vi "AB_820_850_Project_Source_VI.vi"(6 "dataForPrevious":T1, 7 "action":T6, 8 "error in (no error)":errorcluster, 9 "index in":i32, 10 "dataSource in":T5, 11 "buildObject":T4) -> (0 "error out":errorcluster, 1 "index out":i32, 2 "dataSource out":T5, 3 "buildObject out":T4)   [LabVIEW 2020]
doc: "Reads and writes the data to the object property bag."
uses:
  <resource>/Framework/Providers/API/ItemRef.ctl
  <vilib>/AppBuilder/RW_Project/AB_RW_Project_PropBag_Action.ctl
  <vilib>/AppBuilder/RW_Project/AB_RW_Project_Source_Data_for_Previous.ctl
  <vilib>/AppBuilder/AB_BuildType.ctl
  <vilib>/Utility/lvfile.llb/LVFileType.ctl
  <vilib>/Utility/lvfile.llb/NI_FileType.lvlib
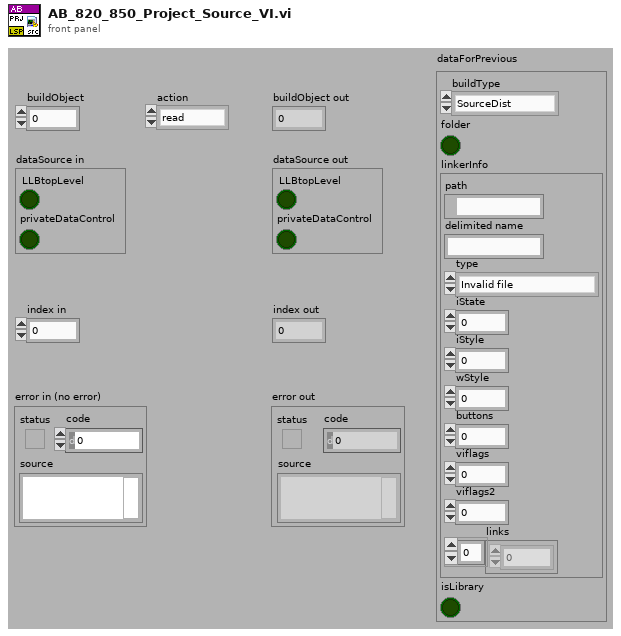
[diagram p1: front panel]
types:
  T1 = typedef "AB_RW_Project_Source_Data_for_Previous.ctl" = cluster{"buildType":T2, "folder":bool, "linkerInfo":cluster{"path":path, "delimited name":string, "type":T3, "iState":u32, "iStyle":u16, "wStyle":u16, "buttons":u16, "viflags":u32, "viflags2":u32, "links":u32[]}, "isLibrary":bool}
  T2 = typedef "AB_BuildType.ctl" = enum16{"SourceDist", "EXE", "DLL", "RTExe"}
  T3 = typedef "NI_FileType.lvlib/LVFileType.ctl" = enum32{"Invalid file", "Unknown type", "Instrument", "Control", "Polymorphic VI", "Project", "Library", "LVClass", "XControl", "XNode", "Shared library", ".NET assembly", "ActiveX interface", "CIN", "Run-time menu", "Palette menu", "Help file", "LLB", "XNode Edit Dependency", "Class Private Data Control", "Statechart", "MathScript .m file", "Ladder Diagram", "LVLibp", "XNode Build Dependency"}
  T4 = typedef "ItemRef.ctl" = u64
  T5 = cluster{"LLBtopLevel":bool, "privateDataControl":bool}
  T6 = typedef "AB_RW_Project_PropBag_Action.ctl" = enum16{"read", "write", "clear", "readPrevious", "writePrevious", "clearPrevious"}
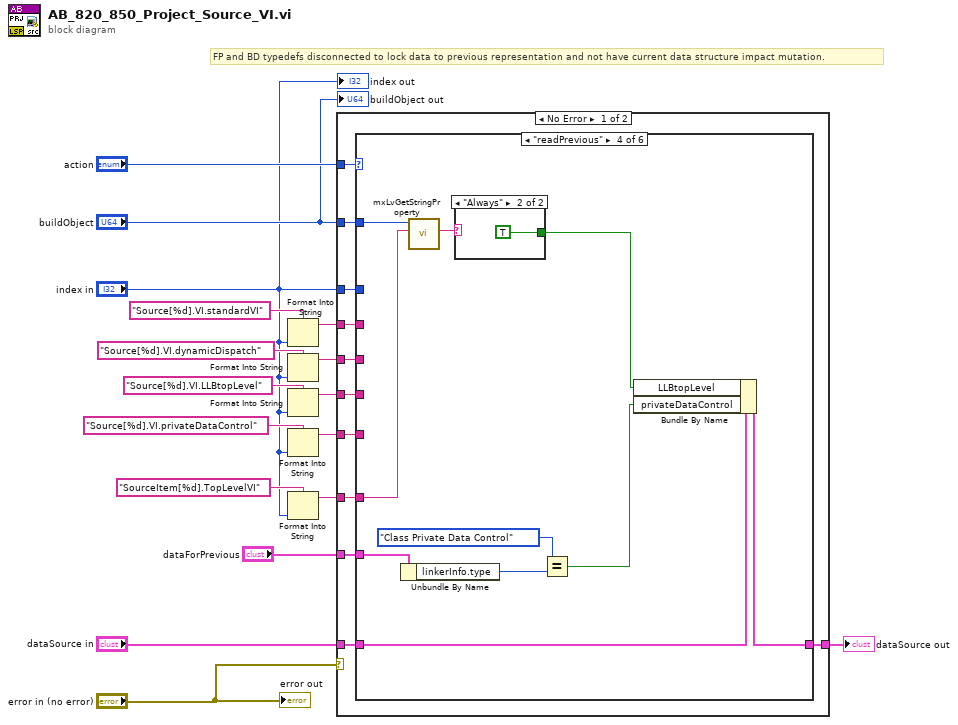
[diagram p0: block diagram]
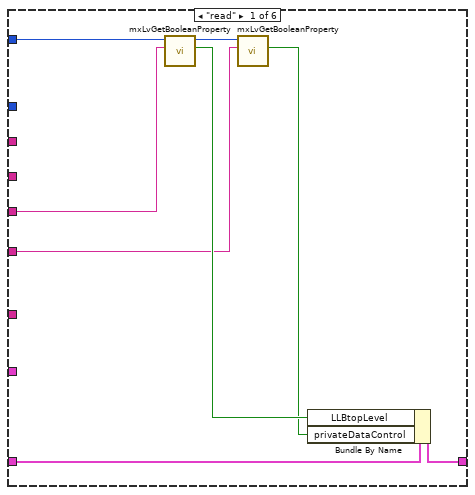
[diagram p2: hidden frame]
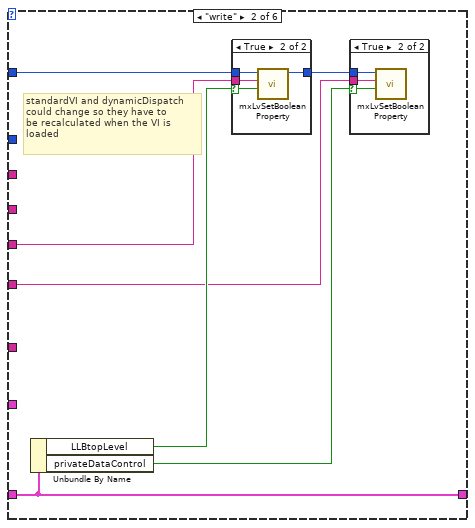
[diagram p3: hidden frame]
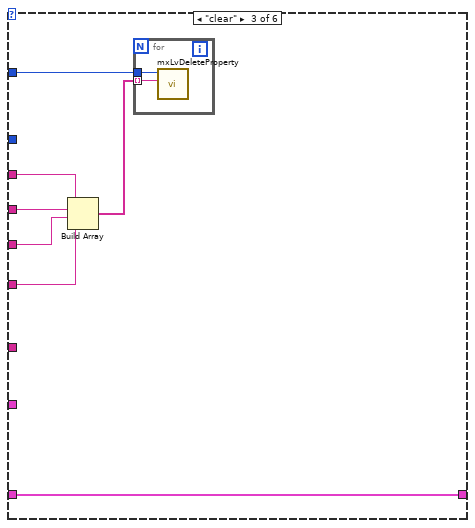
[diagram p6: hidden frame]
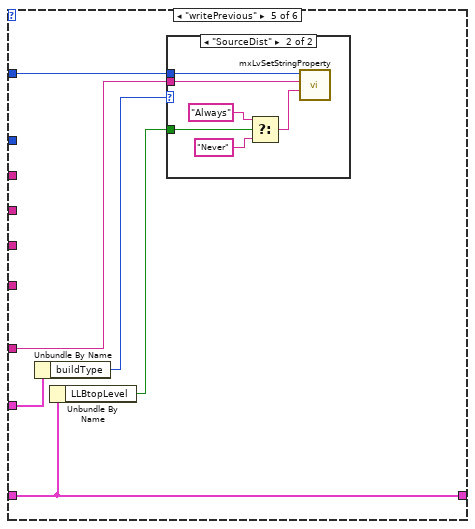
[diagram p8: hidden frame]
diagram:
  # "FP and BD typedefs disconnected to lock data to previous representation and not have current data structure impact mutation."
  n1 = Format Into String(format string="Source[%d].VI.standardVI", "index in") -> (resulting string=w14:string)  [unwired: 2 in, 1 out]
  n2 = Format Into String(format string="Source[%d].VI.dynamicDispatch", "index in") -> (resulting string=w11:string)  [unwired: 2 in, 1 out]
  n3 = Format Into String(format string="Source[%d].VI.LLBtopLevel", "index in") -> (resulting string=w10:string)  [unwired: 2 in, 1 out]
  n4 = Format Into String(format string="Source[%d].VI.privateDataControl", "index in") -> (resulting string=w1:string)  [unwired: 2 in, 1 out]
  n5 = Format Into String(format string="SourceItem[%d].TopLevelVI", "index in") -> (resulting string=w4:string)  [unwired: 2 in, 1 out]
  n6 = case shown="No Error" "error in (no error)" {
    tunnel: "action" -> [w28 _]
    tunnel: "dataSource in" -> [w27 w85]
    tunnel: w14 -> [w26 _]
    tunnel: w11 -> [w25 _]
    tunnel: w10 -> [w24 _]
    tunnel: "index in" -> [w23 _]
    tunnel: [w22 w85] -> w9
    tunnel: "buildObject" -> [w21 _]
    tunnel: "dataForPrevious" -> [w20 _]
    tunnel: w4 -> [w19 _]
    tunnel: w1 -> [w18 _]
    frame No Error {
      n7 = case shown="\"readPrevious\"" w28 {
        tunnel: w21 -> [w32 w42 w53 w69 w75 _]
        tunnel: w27 -> [w36 w43 w58 w70 w76 w84]
        tunnel: w26 -> [_ _ w57 _ _ _]
        tunnel: w25 -> [_ _ w56 _ _ _]
        tunnel: w24 -> [w34 w41 w55 _ _ _]
        tunnel: w23 -> [_ _ _ _ _ _]
        tunnel: [w35 w43 w58 w64 w76 w84] -> w22
        tunnel: w20 -> [_ _ _ w67 w77 _]
        tunnel: w19 -> [_ _ _ w68 w73 _]
        tunnel: w18 -> [w31 w38 w52 _ _ _]
        frame "read" {
          n8 = call <resource>:"mxLvGetBooleanProperty.vi"("Tag"=w34, "Item"=w32) -> ("Value"=w33:bool, "Item"=w30:T4)  [unwired: 7 in, 1 out]
          n9 = call <resource>:"mxLvGetBooleanProperty.vi"("Tag"=w31, "Item"=w30) -> ("Value"=w29:bool)  [unwired: 7 in, 2 out]
          n10 = Bundle By Name(cluster=w36, "LLBtopLevel"=w33, "privateDataControl"=w29) -> (w35:T5)
        }
        frame "write" {
          # "standardVI and dynamicDispatch\ncould change so they have to\nbe recalculated when the VI is\nloaded"
          n11 = Unbundle By Name(w43) -> ("LLBtopLevel"=w40:bool, "privateDataControl"=w37:bool)
          n12 = case shown="True" w40 {
            selector: w40 -> [_ w49]
            tunnel: w42 -> [w47 w51]
            tunnel: w41 -> [_ w50]
            tunnel: [w47 w48] -> w39
            frame False {
            }
            frame True {
              n13 = call <resource>:"mxLvSetBooleanProperty.vi"("Value (F)"=w49, "Tag"=w50, "Item"=w51) -> ("Item"=w48:T4)  [unwired: 7 in, 1 out]
            }
          }
          n14 = case shown="True" w37 {
            selector: w37 -> [_ w44]
            tunnel: w39 -> [_ w46]
            tunnel: w38 -> [_ w45]
            frame False {
            }
            frame True {
              n15 = call <resource>:"mxLvSetBooleanProperty.vi"("Value (F)"=w44, "Tag"=w45, "Item"=w46) -> ()  [unwired: 7 in, 2 out]
            }
          }
        }
        frame "clear" {
          n16 = Build Array(w57, w56, w55, w52) -> (w54:string[])
          n17 = for {
            tunnel: w53 -> [w60]
            tunnel: w54 -> [w59] mode=indexing
            n18 = call <resource>:"mxLvDeleteProperty.vi"("Tag"=w59, "Item"=w60) -> ()  [unwired: 8 in, 2 out]
          }
        }
        frame "readPrevious" {
          n19 = Unbundle By Name(w67) -> ("linkerInfo.type"=w66:T3)
          n20 = call <resource>:"mxLvGetStringProperty.vi"("Tag"=w68, "Item"=w69) -> ("Value"=w62:string)  [unwired: 7 in, 2 out]
          n21 = case shown="\"Always\"" w62 {
            tunnel: [_ TRUE] -> w61
            frame Default {
            }
            frame "Always" {
            }
          }
          n22 = Equal?(x=LVFileType."Class Private Data Control", y=w66) -> (x = y?=w63:bool)
          n23 = Bundle By Name(cluster=w70, "LLBtopLevel"=w61, "privateDataControl"=w63) -> (w64:T5)
        }
        frame "writePrevious" {
          n24 = Unbundle By Name(w77) -> ("buildType"=w74:T2)
          n25 = Unbundle By Name(w76) -> ("LLBtopLevel"=w72:bool)
          n26 = case shown="\"SourceDist\"" w74 {
            tunnel: w75 -> [_ w83]
            tunnel: w73 -> [_ w82]
            tunnel: w72 -> [_ w81]
            frame Default {
            }
            frame "SourceDist" {
              n27 = Select(t="Always", s=w81, f="Never") -> (s? t:f=w78:string)
              n28 = call <resource>:"mxLvSetStringProperty.vi"("Value (\"\")"=w78, "Tag"=w82, "Item"=w83) -> ()  [unwired: 7 in, 2 out]
            }
          }
        }
        frame "clearPrevious" {
        }
      }
    }
    frame Error {
    }
  }
  "dataSource out" <- w9
  "error out" <- "error in (no error)"
  "buildObject out" <- "buildObject"
  "index out" <- "index in"
